vi "Set Throttle.vi"(0 "reference in":refnum<class "Diesel ECU.lvclass">, 5 "Throttle":string, 11 "Error In":errorcluster) -> (4 "reference out":refnum<class "Diesel ECU.lvclass">, 6 "Result":string, 15 "Error Out":errorcluster)   [LabVIEW 2024, in "Diesel ECU.lvclass"]
doc: "Throttle change method implementation"
uses:
  Diesel ECU.lvclass
  Diesel ECU.lvclass/Diesel ECU.ctl
panel:
  # "Connector Pane"
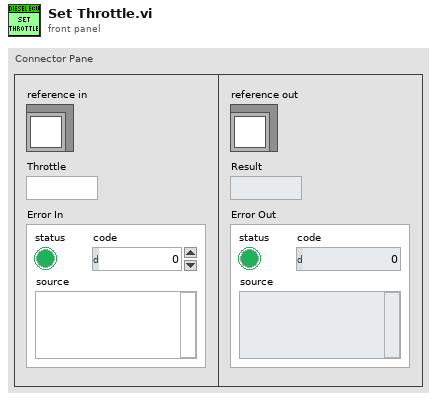
[diagram p1: front panel]
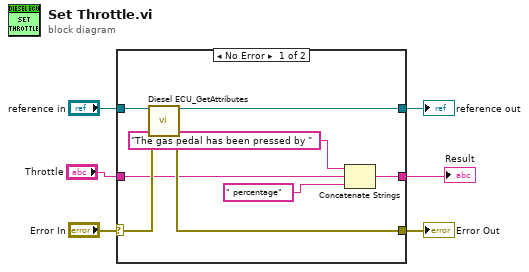
[diagram p0: block diagram]
diagram:
  n1 = case shown="No Error" "Error In" {
    selector: "Error In" -> [w14 w16]
    tunnel: [w13 w16] -> w5
    tunnel: [w11 w15] -> w3
    tunnel: "reference in" -> [w12 w15]
    tunnel: "Throttle" -> [w8 _]
    tunnel: [w7 _] -> w1
    frame No Error {
      n2 = call "Diesel ECU_GetAttributes.vi"("reference in"=w12, "Error In"=w14) -> ("reference out"=w11:refnum<class "Diesel ECU.lvclass">, "Error Out"=w13:errorcluster)  [unwired: 10 in, 2 out]
      n3 = Concatenate Strings("The gas pedal has been pressed by " ("string"), w8, " percentage" ("string")) -> (w7:string)
    }
    frame Error {
    }
  }
  "Error Out" <- w5
  "reference out" <- w3
  "Result" <- w1
